vi "AutoBike FPGA (old).vi"() -> ()   [LabVIEW 2016]
doc: "The roboRIO FPGA Shipping Personality. This personality supports:\n- 8 Analog Input channels with 1 sample\n- 2 Analog Output channels with 1 sample\n- 30 Digital I/O channels with 1 sample\n- 1 RSL channel\n- 4 Relay channels\n- 1 Button\n- 3 LEDs\n- 1 Accelerometer\n- 13 PWM channels\n- 6 Encoder channels\n- 2 SPI channels\n- 2 I2C channels\n- 2 UART channels\n- 1 CAN channel\n- 2 Analog Input Interrupt\n- 5 Digital Input Interrupt\n- 1 Timer Interrupt"
uses:
  Sub VIs for FPGA/SubVIs needed for the customize FPGA VI/Utilities/Start Boolean.ctl
  <vilib>/rvi/Analysis/control/PID/Typedef/niFpgaPID_OutputRange.ctl
  <vilib>/rvi/Analysis/control/PID/Typedef/niFpgaPID_PIDGains.ctl
  <vilib>/rvi/Analysis/control/PID/Typedef/niFpgaPID_PIGains.ctl
  <vilib>/Platform/TimedLoop/XDataNode/timing_clust.ctl
  <vilib>/Platform/TimedLoop/XDataNode/nitl_modes.ctl
  <vilib>/Platform/TimedLoop/XDataNode/wakeup.ctl
  <vilib>/rvi/Analysis/control/PID/Typedef/niFpgaPID_SetpointWeightings.ctl
  <vilib>/rvi/Emulation/niFpgaGetClockAttributes.vi
  <vilib>/rvi/Emulation/niFpgaSctlEmulationGetInTimedLoop.vi
  <vilib>/rvi/Emulation/niFpgaEmulationReportErrorSimple.vi
  <vilib>/rvi/eio/common/nirviEmuTemplateMethod_errors.vi
  <vilib>/rvi/Emulation/niFpgaCriticalErrorInLSC.vi
  <vilib>/rvi/Emulation/niFpgaProcessEmulError.vi
  <vilib>/rvi/Emulation/niFpgaEmulationIsFPGAContextNoSignature.vi
  <vilib>/rvi/errors/niFpgaSetErrorForExecOnDevCompSimple.vi
  <vilib>/rvi/eio/common/nirviEmuReportErrorAndStop.vi
  <vilib>/rvi/DataTransferAndStorage/Container/Common/niFpgaContainerGetUniqueNameForEmu.vi
  <vilib>/rvi/FIFO/Fifo_Resource/nirvififoEmulationSetSize.vi
  <vilib>/rvi/FIFO/Fifo_Resource/nirviFifoEmulationQueueMgr.vi
  <instcachedir>/0/nirviFifoEmulationQueueMgr_E5CAEC123FF24DC58D834DCA3CDAA9B5.lvgen/nirviFifoEmulationQueueMgr_E5CAEC123FF24DC58D834DCA3CDAA9B5_002.vi
  <vilib>/Utility/error.llb/Clear Errors.vi
  <vilib>/rvi/FIFO/Fifo_Resource/nirvififoEmulationCreateLock.vi
  <vilib>/rvi/FIFO/Fifo_Resource/nirvififoEmulationObtainLock.vi
  <vilib>/rvi/FIFO/Fifo_Resource/nirvififoEmulationReleaseLock.vi
  <vilib>/rvi/occurrence/nirviWaitOnOccurrenceBase.vi
  <vilib>/rvi/errors/nirviReportUnexpectedCaseInternalError.vi
  <vilib>/rvi/errors/nirviReportUnexpectedCaseInternalError (U32).vi
  <vilib>/rvi/FIFO/Fifo_Resource/nirvififoEmulationDetermineInputValidOut.vi
  <vilib>/rvi/Analysis/control/PID/SubVIs/niFpgaPID_PIWrapper.vi
  <vilib>/rvi/Analysis/control/PID/SubVIs/niFpgaPID_PIDWrapper.vi
  <vilib>/rvi/DataTransferAndStorage/Container/Common/niFpgaContainerSetEmuInfo.vi
  <vilib>/eio/EIONode/EIONode.xnode
  <vilib>/rvi/DataTransferAndStorage/Container/XNode/niFpgaContainer.xnode
  <vilib>/rvi/FIFO/Fifo_Resource/nirvififoEmulationRead.vi
  <vilib>/rvi/FIFO/Fifo_Resource/nirvififoEmulationWrite.vi
  <vilib>/Platform/TimedLoop/XDataNode/XDataNode.xnode
  <vilib>/rvi/LocalResourceManager/LocalResourceManager.xnode
  <vilib>/Platform/TimedLoop/XDataNode/XDNodeRunTimeDep.lvlib
panel:
  out "Value Channel 3":i32
  out "Value Channel 2":i32
  in  "Speed output range":T1={"output high (Inf)"=0.0001, "output low (-Inf)"=-0.0001}
  in  "PI gains":T2={"proportional gain"=40.0, "integral gain"=15.0} {"proportional gain" step=0.125}
  out "Steering loop time":u32
  in  "Steering motor on?":bool
  in  "Gain Sch, on?":bool
  in  "Gain Sch.":T3[](array[typedef])=[{"proportional gain"=0.0, "integral gain"=0.0, "derivative gain"=0.0, "filter coefficient"=0.0}, {"proportional gain"=0.0, "integral gain"=0.0, "derivative gain"=0.0, "filter coefficient"=0.0}, {"proportional gain"=0.0, "integral gain"=0.0, "derivative gain"=0.0, "filter coefficient"=0.0}, {"proportional gain"=0.0, "integral gain"=0.0, "derivative gain"=0.0, "filter coefficient"=0.0}] {"filter coefficient" min=0 max=1; "proportional gain" step=0.125}
  in  "output range Sch.":T1[](array[typedef])=[{"output high (Inf)"=0.0, "output low (-Inf)"=0.0}, {"output high (Inf)"=0.0, "output low (-Inf)"=0.0}, {"output high (Inf)"=0.0, "output low (-Inf)"=0.0}, {"output high (Inf)"=0.0, "output low (-Inf)"=0.0}]
  in  "Desired steering angle":sgl format="%#_13g"
  in  "Stop PID controller":bool
  in  "Pid reset (F)":bool
  out "Current steering angle":sgl
  out "Duty cycle (steering)":sgl
  out "Position 2":i64
  in  "LQR Duty Cycle":sgl
  in  "LQR Direction":bool
  in  "Shut Down BW":bool
  out "Current speed":sgl
  out "Duty cycle (BW)":sgl
  in  "Reference speed in km/h":sgl=15.0
  out "Filtered data":i32
  out "Value Channel 0":i32
  out "Channel 4 position":u8
  out "Channel 5 position":u8
  out "Channel 6 position":u8
  out "Channel 7 position":u8
  out "Position":i32
  in  "Stop encoder":bool
  in  "Reset counter":bool
  in  "Stop direction switch":bool
  in  "Direction":bool
  out "HallSensorValue":u8
  out "dt":u32
  out "DIO.SPI_CS3:0.IN":u8 format="%08b"
  in  "DIO.SPI_CS3:0.DIR":u8 format="%08b"
  in  "DIO.SPI_CS3:0.OUT":u8 format="%08b"
  in  "IRQ.TIMER.SETTIME":T4
  in  "IRQ.TIMER.WRITE":u32
  out "IRQ.TIMER.READ":u32
  in  "IRQ.DI_BTN.NO":u8
  in  "IRQ.DI_BTN.CNT":u32
  in  "IRQ.DI_BTN.FALL":bool
  in  "IRQ.DI_BTN.RISE":bool
  in  "IRQ.DI_BTN.ENA":bool
  in  "IRQ.AI_B_0.HYSTERESIS":u16=17
  in  "IRQ.AI_B_1.HYSTERESIS":u16=17
  in  "IRQ.AI_B_1.NO":u8
  in  "IRQ.AI_B_0.NO":u8
  in  "IRQ.AI_B_1.THRESHOLD":u16
  in  "IRQ.AI_B_0.THRESHOLD":u16
  in  "IRQ.AI_B_3:0.CNFG":u8 format="%.0b"
  in  "IRQ.DIO_B_0.NO":u8
  in  "IRQ.DIO_B_1.NO":u8
  in  "IRQ.DIO_B_2.NO":u8
  in  "IRQ.DIO_B_3.NO":u8
  in  "IRQ.DIO_B_3.CNT":u32
  in  "IRQ.DIO_B_2.CNT":u32
  in  "IRQ.DIO_B_1.CNT":u32
  in  "IRQ.DIO_B_0.CNT":u32
  in  "IRQ.DIO_B_7:0.FALL":u8 format="%08b"
  in  "IRQ.DIO_B_7:0.RISE":u8 format="%08b"
  in  "IRQ.DIO_B_7:0.ENA":u8 format="%08b"
  in  "SPI.SPI.IRQ.NO":u8=15
  in  "SPI.B.IRQ.NO":u8=15
  out "DIO.DIO_9:8.IN":u8 format="%08b"
  in  "ENC.DIO_3.CNFG":u8 format="%08b"
  out "ENC.DIO_3.CNTR":u32
  out "ENC.DIO_3.STAT":u8 format="%08b"
  in  "ENC.DIO_4.CNFG":u8 format="%08b"
  out "ENC.DIO_4.CNTR":u32
  out "ENC.DIO_4.STAT":u8 format="%08b"
  in  "DIO.DIO_9:8.OUT":u8 format="%08b"
  in  "DIO.DIO_9:8.DIR":u8 format="%08b"
  in  "ENC.DIO_2.CNFG":u8 format="%08b"
  out "ENC.DIO_2.CNTR":u32
  out "ENC.DIO_2.STAT":u8 format="%08b"
  out "ENC.DIO_1.STAT":u8 format="%08b"
  out "ENC.DIO_1.CNTR":u32
  in  "ENC.DIO_1.CNFG":u8 format="%08b"
  out "DIO.DIO_7:0.IN":u8 format="%08b"
  in  "SYS.SELECTDIO":u8 format="%08b"
  in  "DIO.DIO_7:0.DIR":u8 format="%08b"
  in  "DIO.DIO_7:0.OUT":u8 format="%08b"
  out "ENC.DIO_0.STAT":u8 format="%08b"
  out "ENC.DIO_0.CNTR":u32
  in  "ENC.DIO_0.CNFG":u8 format="%08b"
  out "DI.BTN":u8 format="%08b"
  in  "DO.LED 5:0":u8 format="%06b"
  in  "DO.RSL.OUT":bool
  out "SPI.SPI.STAT":u8 format="%08b"
  in  "SPI.SPI.GO":T4
  in  "SPI.SPI.CNT":u16
  in  "SPI.SPI.CNFG":u16 format="%016b"
  out "SPI.SPI.DATI":u16
  in  "SPI.SPI.DATO":u16
  out "I2C.I2C.DATI":u8
  out "I2C.I2C.STAT":u8 format="%08b"
  in  "I2C.I2C.DATO":u8
  in  "I2C.I2CADDR":u8 format="%08b"
  in  "I2C.I2C.CNTR":u8
  in  "I2C.I2C.CNTL":u8 format="%08b"
  in  "I2C.I2C.CNFG":u8 format="%08b"
  in  "I2C.I2C.GO":T4
  out "ACC.Z.VAL":u16
  out "ACC.Y.VAL":u16
  out "ACC.X.VAL":u16
  in  "DO.RELAY.OUT":u8 format="%08b"
  out "SYS.ACC.RDY":bool
  out "SYS.RDY":bool
  in  "PWM.PWM_5.MAX":u16
  in  "PWM.PWM_5.CMP":u16
  in  "PWM.PWM_5.CNFG":u8 format="%08b"
  in  "PWM.PWM_5.CS":u8
  out "PWM.PWM_5.CNTR":u16
  in  "PWM.PWM_6.MAX":u16
  in  "PWM.PWM_6.CMP":u16
  in  "PWM.PWM_6.CNFG":u8 format="%08b"
  in  "PWM.PWM_6.CS":u8
  out "PWM.PWM_6.CNTR":u16
  in  "PWM.PWM_7.MAX":u16
  in  "PWM.PWM_7.CMP":u16
  in  "PWM.PWM_7.CNFG":u8 format="%08b"
  in  "PWM.PWM_7.CS":u8
  out "PWM.PWM_7.CNTR":u16
  in  "PWM.PWM_8.MAX":u16
  in  "PWM.PWM_8.CMP":u16
  in  "PWM.PWM_8.CNFG":u8 format="%08b"
  in  "PWM.PWM_8.CS":u8
  out "PWM.PWM_8.CNTR":u16
  in  "PWM.PWM_9.MAX":u16
  in  "PWM.PWM_9.CMP":u16
  in  "PWM.PWM_9.CNFG":u8 format="%08b"
  in  "PWM.PWM_9.CS":u8
  out "PWM.PWM_9.CNTR":u16
  in  "PWM.PWM_4.MAX":u16
  in  "PWM.PWM_4.CMP":u16
  in  "PWM.PWM_4.CNFG":u8 format="%08b"
  in  "PWM.PWM_4.CS":u8
  out "PWM.PWM_4.CNTR":u16
  in  "PWM.PWM_3.MAX":u16
  in  "PWM.PWM_3.CMP":u16
  in  "PWM.PWM_3.CNFG":u8 format="%08b"
  in  "PWM.PWM_3.CS":u8
  out "PWM.PWM_3.CNTR":u16
  in  "PWM.PWM_2.MAX":u16
  in  "PWM.PWM_2.CMP":u16
  in  "PWM.PWM_2.CNFG":u8 format="%08b"
  in  "PWM.PWM_2.CS":u8
  out "PWM.PWM_2.CNTR":u16
  in  "PWM.PWM_1.MAX":u16
  in  "PWM.PWM_1.CMP":u16
  in  "PWM.PWM_1.CNFG":u8 format="%08b"
  in  "PWM.PWM_1.CS":u8
  out "PWM.PWM_1.CNTR":u16
  out "PWM.PWM_0.CNTR":u16
  in  "PWM.PWM_0.CS":u8
  in  "PWM.PWM_0.CNFG":u8 format="%08b"
  in  "PWM.PWM_0.CMP":u16
  in  "PWM.PWM_0.MAX":u16
  in  "AO.B_0.VAL":u16
  in  "AO.B_1.VAL":u16
  in  "AO.SYS.GO":T4
  out "AO.SYS.STAT":bool
  out "AI.B_0.VAL":u16
  out "AI.B_1.VAL":u16
  out "AI.B_2.VAL":u16
  out "AI.B_3.VAL":u16
  out "AI.AI_0.VAL":u16
  out "AI.AI_1.VAL":u16
  out "AI.AI_2.VAL":u16
  out "AI.AI_3.VAL":u16
  out "SYS.AI.RDY":bool
  in  "SYS.SELECTB":u8 format="%08b"
  in  "DIO.B_7:0.OUT":u8 format="%08b"
  in  "DIO.B_7:0.DIR":u8 format="%08b"
  out "DIO.B_7:0.IN":u8 format="%08b"
  in  "DIO.B_15:8.OUT":u8 format="%08b"
  in  "DIO.B_15:8.DIR":u8 format="%08b"
  out "DIO.B_15:8.IN":u8 format="%08b"
  in  "SPI.B.DATO":u16
  out "SPI.B.DATI":u16
  in  "SPI.B.CNFG":u16 format="%016b"
  in  "SPI.B.CNT":u16
  in  "SPI.B.GO":T4
  out "SPI.B.STAT":u8 format="%08b"
  in  "PWM.B_0.MAX":u16
  in  "PWM.B_0.CMP":u16
  in  "PWM.B_0.CNFG":u8 format="%08b"
  in  "PWM.B_0.CS":u8
  out "PWM.B_0.CNTR":u16
  in  "PWM.B_1.CMP":u16
  in  "PWM.B_1.MAX":u16
  out "PWM.B_1.CNTR":u16
  in  "PWM.B_1.CNFG":u8 format="%08b"
  in  "PWM.B_1.CS":u8
  in  "PWM.B_2.CMP":u16
  in  "PWM.B_2.MAX":u16
  out "PWM.B_2.CNTR":u16
  in  "PWM.B_2.CNFG":u8 format="%08b"
  in  "PWM.B_2.CS":u8
  in  "I2C.B.DATO":u8
  out "I2C.B.DATI":u8
  in  "I2C.B.ADDR":u8 format="%08b"
  in  "I2C.B.CNTR":u8
  in  "I2C.B.CNTL":u8 format="%08b"
  out "I2C.B.STAT":u8 format="%08b"
  in  "I2C.B.CNFG":u8 format="%08b"
  in  "I2C.B.GO":T4
  in  "ENC.B.CNFG":u8 format="%08b"
  out "ENC.B.CNTR":u32
  out "ENC.B.STAT":u8 format="%08b"
  # "System"
  # "Onboard Devices"
  # "Connector B"
  # "DIO"
  # "SPI"
  # "PWM"
  # "I2C"
  # "AI"
  # "RELAY"
  # "RSL"
  # "Accelerometer"
  # "SPI Master"
  # "Analog Input"
  # "Analog Output"
  # "Digital I/O"
  # "Counters / PWM"
  # "Digital I/O"
  # "Encoders"
  # "IO Configuration"
  # "Buttons & LEDs"
  # "SPI CS DIO"
  # "Analog Interrupt"
  # "Digital Interrupt"
  # "Encoders"
  # "IO Configuration"
  # "Button Interrupt"
  # "I2C Master"
  # "FPGA Timer"
types:
  T1 = typedef "niFpgaPID_OutputRange.ctl" = cluster{"output high (Inf)":sgl, "output low (-Inf)":sgl}
  T2 = typedef "niFpgaPID_PIGains.ctl" = cluster{"proportional gain":sgl, "integral gain":sgl}
  T3 = typedef "niFpgaPID_PIDGains.ctl" = cluster{"proportional gain":sgl, "integral gain":sgl, "derivative gain":sgl, "filter coefficient":sgl}
  T4 = typedef "Start Boolean.ctl" = bool
  T5 = typedef "XDNodeRunTimeDep.lvlib/timing_clust.ctl" = cluster{"Expected End [f-1]":u64, "Actual End [f-1]":u64, "Finished Late? [f-1]":bool, "Expected End [i-1]":u64, "Actual End [i-1]":u64, "Finished Late? [i-1]":bool, "Expected Start [i]":u64, "Actual Start [i]":u64, "Expected Start [f]":u64, "Actual Start [f]":u64, "Source Name":string, "Structure Name":string, "Period":i64, "Deadline":i64, "Offset":i64, "Start":i64, "Priority":i32, "Timeout":i32, "Mode":T6, "Wakeup Reason":T7, "Error":errorcluster, "Source Type":string, "Secondary Source Type":string, "Global End Time":u64, "Global Start Time":u64, "Frame Duration":u64, "Iteration Duration":u64, "Assigned CPU":i32, "I/O Scan Engine Mode":u32}
  T6 = typedef "XDNodeRunTimeDep.lvlib/nitl_modes.ctl" = enum32{"No Change", "Process missed periods, maintain original phase", "Discard missed periods, maintain original phase", "Process missed periods, ignore original phase", "Discard missed periods, ignore original phase"}
  T7 = typedef "XDNodeRunTimeDep.lvlib/wakeup.ctl" = enum32{"Normal", "Aborted", "Asynchronous wakeup", "Timing source error", "Timed loop error", "Timeout"}
  T8 = typedef "niFpgaPID_SetpointWeightings.ctl" = cluster{"proportional weighting (1)":sgl, "derivative weighting (0)":sgl}
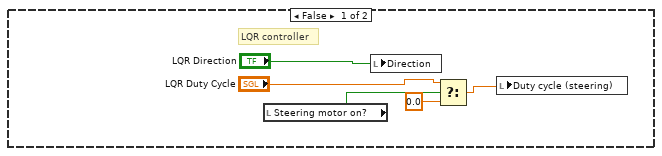
[diagram p8: hidden frame]
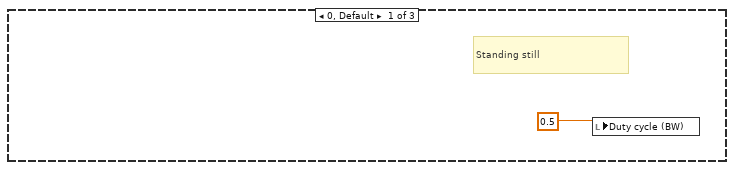
[diagram p9: hidden frame]
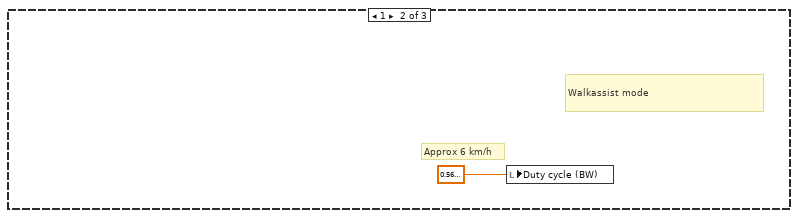
[diagram p10: hidden frame]
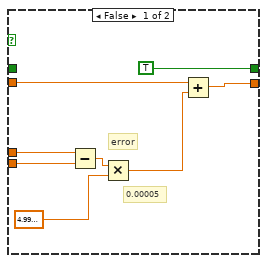
[diagram p11: hidden frame]
diagram:
  # "Runs at 40 MHz"
  # "The accelerometer nodes take some time before the FPGA can first read the values. This is because it takes time to read from the accelerometer. An iteration of the While Loop will not complete until the accelerometer values have been read.\n\nAfter the completion of the first iteration of the While Loop, all indicators have valid values."
  # "The analog output nodes take some time before the FPGA write the values to the pins. The GO and STAT registers are used to handshake between the FPGA and host. When the host wants the values to be written, the host sets the GO register to TRUE. If the host reads the STAT register before setting the value of the GO register, it can wait for the value of the STAT register to invert. The value inversion tells the host that the output values have been written."
  # "The FPGA timer fires the interrupt request (IRQ) when TIMER.Read counts down to zero. If TIMER.Read is not zero, it counts down to one per microsecond."
  # "The analog input nodes take some time before the FPGA can first read the values. This is because it takes time to set up the Analog-to-Digital converter (ADC) and convert the first reading. An iteration of the While Loop will not complete until all the analog input channels have been sampled.\n\nAfter the completion of the first iteration of the While Loop, all indicators have valid values."
  # "Note: On some hardware a \"ghosting effect\" may occur on any unconnected AI channels. For example, if channel AI0 is connected and channels AI1~AI7 are not connected the the value read at AI0 may be seen on indicators AI1~AI7. This is common for hardware that use a multiplexed (MUXed) Analog-to-Digital converter (ADC), because the input analog signal is used to charge a capacitor which does not discharge before the unconnected channel is read.\n\nYou can hide the \"ghosting effect\" by using an mask register. This register is used to decide when the indicator should be updated."
  # "The only interface that sends interrupts to the RT side. Timer interrupts, analog input interrupts, digital input interrupts, and SPI interrupt share this interface.\n\nAll interrupts work in sequence. One interrupt waits until the previous interrupt request (IRQ) gets acknowledged on the RT side."
  # "NOTE: The SYS.RDY boolean MUST exist and must become TRUE at some point otherwise the myRIO API will not function correctly."
  # "There is some delay between when the FPGA code starts and the analog inputs, accelerometer, and scaling values outputs are valid. If the host wants to ensure that there are valid values in theses registers it should wait for each subsystem to finish its initialization process. \n\nWhen all subsystems have finished initializinig, the SYS.RDY indicator will be true, which can be polled by the host to determine the status of the FPGA. Alternatively, the host can poll the individual SYS.xx.RDY indicators to determine the status of the individual subsystems.\n\nThis loop continues indefinitely, essentially making SYS.RDY a read-only register."
  n1 = while {
    shift-right: [w32] -> _
    shift-left: TRUE ("DIO/DIO3") -> [w33]
    stop <- FALSE stop-if-true
    n2 = flat-sequence {
      tunnel: w33 -> [w36]
      tunnel: [w36] -> w31
      tunnel: [u8 0] -> w30
      tunnel: [w34] -> w29
      tunnel: w31 -> [w41]
      tunnel: w30 -> [w39]
      tunnel: w29 -> [w38]
      tunnel: [w40] -> w28
      tunnel: [w37] -> w27
      tunnel: [w63] -> w32
      tunnel: w28 -> [w63]
      tunnel: [w62] -> w26
      tunnel: w27 -> [w60]
      frame #0 {
        n3 = call "Tick Count4"() -> ("Tick Count(uSec)"=w34:u32)
      }
      frame #1 {
        n4 = node-c288() -> (w43:T5)  [unwired: 1 in]
        n5 = timed-loop {
          shift-right: [w44] -> _
          shift-left: w39 -> [w45]
          shift-right: [w52] -> w40
          shift-left: w41 -> [w55]
          timing: w43 -> [_]
          timing-out: [_] -> w42
          tunnel: w38 -> [w54]
          tunnel: [w54] -> w37
          stop <- w47 stop-if-true
          # "Calculates the time it takes to collect 2 rises, i.e one magnet"
          # "Reads the output from the hallsensor and outputs the number of change in rises"
          # "Hallsensor counter"
          n6 = xnode "FPGA I/O Node"() -> ("DIO/DIO8"=w52:bool)  [unwired: 1 in, 1 out]
          n7 = Exclusive Or(1:w55, 2:w52) -> (0:w50:bool)
          n8 = Not And(1:TRUE ("y"), 2:w52) -> (0:w51:bool)
          n9 = And(x=w51, y=w50) -> (x .and. y?=w49:bool)
          n10 = Increment(x=w45) -> (x+1=w48:u8)
          n11 = Select(t=w48, s=w49, f=w45) -> (s? t:f=w44:u8)
          "HallSensorValue" <- w44
          n12 = Equal?(x=u8 2, y=w44) -> (x = y?=w47:bool)
        }
        n13 = node-c288(w42) -> ()
      }
      frame #2 {
        n14 = call "Tick Count"() -> ("Tick Count(uSec)"=w61:u32)
        n15 = Subtract(x=w61, y=w60) -> (x-y=w62:u32)
      }
    }
    n16 = To Long Integer(number=w26) -> (32bit integer=w25:i32)
    n17 = call "Median filter.vi"("Rawdata"=w25) -> ("Filtered element"=w22:i32)  [unwired: 10 in]
    n18 = Equal To 0?(x=w22) -> (x = 0?=w24:bool)
    n19 = Select(t=1, s=w24, f=w22) -> (s? t:f=→"Filtered data":i32)
  }
  n20 = node-c288() -> (w8:T5)  [unwired: 1 in]
  n21 = while {
    stop <- FALSE stop-if-true
    # "PWM signal to backwheel motor"
    n22 = flat-sequence {
      tunnel: [w69] -> w65
      tunnel: w65 -> [w72]
      frame #0 {
        # "80 000ticks=500Hz"
        n23 = call "Loop Timer2"("Count(Ticks)"=u32 80000) -> ()  [unwired: 1 out]
      }
      frame #1 {
        n24 = local read "Duty cycle (BW)"() -> (w67:sgl)
        n25 = xnode "FPGA I/O Node"("PWM/PWM8"=TRUE) -> ()  [unwired: 1 in, 1 out]
        n26 = Multiply(x=w67, y=sgl 80000.0) -> (x*y=w70:sgl)
        n27 = To Unsigned Long Integer(number=w70) -> (unsigned 32bit integer=w69:u32)
      }
      frame #2 {
        n28 = call "Wait2"("Count(Ticks)"=w72) -> ()  [unwired: 1 out]
      }
      frame #3 {
        n29 = xnode "FPGA I/O Node"("PWM/PWM8"=FALSE) -> ()  [unwired: 1 in, 1 out]
      }
    }
  }
  n30 = node-c288() -> (w6:T5)  [unwired: 1 in]
  n31 = while {
    stop <- FALSE stop-if-true
    # "Host Synchronization"
    n32 = local read "SYS.ACC.RDY"() -> (w75:bool)
    n33 = local read "SYS.AI.RDY"() -> (w77:bool)
    n34 = Compound Arithmetic op=AND(w77, w75) -> (→"SYS.RDY":bool)
  }
  n35 = timed-loop {
    shift-right: [w88] -> _
    shift-left: 0 -> [w79]
    shift-right: [w85] -> _
    shift-left: _ -> [w83]
    shift-right: [w84] -> _
    shift-left: _ -> [w82]
    timing: w8 -> [_]
    timing-out: [_] -> w7
    stop <- "Stop encoder" stop-if-true
    # "Decoder, reads both signals and check if there is any change to any of the channels, if there is a change current A channel\nis compared to previous B channel to determine which direction the motor is going and updates the position counter\naccordingly. The counter is resetted each time the Main VI is deployed."
    # "Steering motor decoder"
    n36 = xnode "FPGA I/O Node"() -> ("DIO/DIO0"=w85:bool, "DIO/DIO1"=w84:bool)  [unwired: 2 in, 2 out]
    n37 = Exclusive Or(1:w82, 2:w85) -> (0:w81:bool)
    n38 = Select(t=0, s="Reset counter", f=w79) -> (s? t:f=w87:i32)
    n39 = Exclusive Or(1:w83, 2:w85) -> (0:w95:bool)
    n40 = Exclusive Or(1:w82, 2:w84) -> (0:w94:bool)
    n41 = Or(x=w95, y=w94) -> (x .or. y?=w80:bool)
    n42 = Select(t=1, s=w81, f=-1) -> (s? t:f=w90:i32)
    n43 = Add(x=w90, y=w87) -> (x+y=w89:i32)
    n44 = Select(t=w89, s=w80, f=w87) -> (s? t:f=w88:i32)
    "Position" <- w88
  }
  n45 = timed-loop {
    timing: w6 -> [_]
    timing-out: [_] -> w5
    stop <- "Stop direction switch" stop-if-true
    # "Switch the direction of the steering\nmotor."
    # "Switch direction"
    n46 = xnode "FPGA I/O Node"("DIO/DIO2"="Direction") -> ()  [unwired: 1 in, 1 out]
  }
  n47 = while {
    stop <- FALSE stop-if-true
    # "PWM signal to steering motor"
    n48 = flat-sequence {
      tunnel: [w105] -> w102
      tunnel: [w110] -> w104
      tunnel: w102 -> [w107]
      tunnel: w104 -> [w112]
      frame #0 {
        w105 = u32 40000 ("Freq")
        # "40000 ticks=1kHz"
        n49 = call "Loop Timer3"("Count(Ticks)"=w105) -> ()  [unwired: 1 out]
      }
      frame #1 {
        # "Too make sure 0 duty \ncycle is generated"
        n50 = local read "Duty cycle (steering)"() -> (w108:sgl)
        n51 = To Single Precision Float(number=w107) -> (single precision float=w106:sgl)
        n52 = Not Equal To 0?(x=w108) -> (x != 0?=w109:bool)
        n53 = Multiply(x=w108, y=w106) -> (x*y=w111:sgl)
        n54 = xnode "FPGA I/O Node"("PWM/PWM0"=w109) -> ()  [unwired: 1 in, 1 out]
        n55 = To Unsigned Long Integer(number=w111) -> (unsigned 32bit integer=w110:u32)
      }
      frame #2 {
        n56 = call "Wait3"("Count(Ticks)"=w112) -> ()  [unwired: 1 out]
      }
      frame #3 {
        n57 = xnode "FPGA I/O Node"("PWM/PWM0"=FALSE ("PWM/PWM8")) -> ()  [unwired: 1 in, 1 out]
      }
    }
  }
  n58 = while {
    stop <- FALSE stop-if-true
    # "Convert Hall sensor pulses to current speed"
    n59 = local read "Filtered data"() -> (w115:i32)
    n60 = call "Speed conversion.vi"("Filtered data"=w115) -> ("Numeric"=→"Current speed":sgl)  [unwired: 10 in]
  }
  n61 = node-c288(w5) -> ()
  n62 = while {
    stop <- FALSE stop-if-true
    # "Backwheel motor control"
    n63 = local read "Channel 5 position"() -> (w117:u8)
    n64 = case shown="2" w117 {
      frame 0, Default {
        # "Standing still"
        n65 = local write "Duty cycle (BW)"(sgl 0.5 ("Duty cycle out 2")) -> ()
      }
      frame 1 {
        # "Walkassist mode"
        # "Approx 6 km/h"
        n66 = local write "Duty cycle (BW)"(sgl 0.56 ("Duty cycle out")) -> ()
      }
      frame 2 {
        n67 = while {
          shift-right: [w125] -> _
          shift-left: sgl 0.56 -> [w135]
          shift-right: [w134] -> _
          shift-left: _ -> [w133]
          stop <- w136 stop-if-true
          w124 = sgl 3.0 ("upper limit")
          # "P or PI controller"
          # "Cruise control"
          n68 = local read "Current speed"() -> (w123:sgl)
          n69 = Subtract(x="Reference speed in km/h", y=w123) -> (x-y=w131:sgl)
          n70 = Negate(x=w124) -> (-x=w129:sgl)
          n71 = In Range and Coerce(upper limit=w124, x=w131, lower limit=w129) -> (In Range?=w130:bool)  [unwired: 1 out]
          n72 = case shown="True" w130 {
            tunnel: [w146 w155] -> w128
            tunnel: "Reference speed in km/h" -> [w142 w153]
            tunnel: w135 -> [w144 w154]
            tunnel: w123 -> [w141 w152]
            tunnel: [TRUE FALSE] -> w134
            tunnel: w133 -> [_ w147]
            frame False {
              # "error"
              # "0.00005"
              n73 = Subtract(x=w142, y=w141) -> (x-y=w143:sgl)
              n74 = Multiply(x=w143, y=sgl 5e-05 ("P gain")) -> (x*y=w145:sgl)
              n75 = Add(x=w144, y=w145) -> (x+y=w146:sgl)
            }
            frame True {
              # "Gains"
              # "Output range"
              n76 = call-poly <vilib>:"niFpgaPID_Wrapper.vi"("setpoint"=w153, "reset? (F)"=w147, "process variable"=w152, "gains"="PI gains", "output range"="Speed output range") -> ("output"=w151:sgl)  [unwired: 8 in, 2 out]
              n77 = Add(x=w154, y=w151) -> (x+y=w155:sgl)
            }
          }
          n78 = local read "Channel 5 position"() -> (w138:u8)
          n79 = In Range and Coerce(upper limit=sgl 1.0, x=w128, lower limit=sgl 0.565) -> (coerced(x)=w125:sgl)  [unwired: 1 out]
          "Duty cycle (BW)" <- w125
          n80 = Not Equal?(x=w138, y=u8 2) -> (x != y?=w136:bool)
          n81 = call "Loop Timer5"("Count(Ticks)"=u32 400000 ("Speed loop time")) -> ()  [unwired: 1 out]
        }
      }
    }
  }
  n82 = while {
    stop <- FALSE stop-if-true
    # "Interrupt to RT"
    n83 = xnode ("FIFO Method Node")("Timeout"=-1) -> ("Element"=w158:u8)  [unwired: 1 in, 2 out]
    n84 = call <vilib>:"niFPGA Interrupt.vi"("Wait Until Cleared (F)"=TRUE, "IRQ Number (0)"=w158) -> ()  [unwired: 1 in]
  }
  n85 = while {
    stop <- FALSE stop-if-true
    # "RC steering motor switch"
    n86 = local read "Channel 6 position"() -> (w161:u8)
    n87 = Greater Than 0?(x=w161) -> (x > 0?=w160:bool)
    n88 = case shown="True" w160 {
      frame False {
        # "LQR controller"
        n89 = local read "Steering motor on?"() -> (w164:bool)
        n90 = local write "Direction"("LQR Direction") -> ()
        n91 = Select(t="LQR Duty Cycle", s=w164, f=sgl 0.0) -> (s? t:f=w165:sgl)
        n92 = local write "Duty cycle (steering)"(w165) -> ()
      }
      frame True {
        # "Control loop"
        n93 = while {
          shift-right: [w172] -> _
          shift-left: u32 0 ("Tick Count(Ticks)") -> [w173]
          stop <- w183 stop-if-true
          n94 = local read "Position"() -> (w186:i32)
          n95 = To Single Precision Float(number=w186) -> (single precision float=w185:sgl)
          n96 = call "Tick Count2"() -> ("Tick Count(Ticks)"=w172:u32)
          n97 = call "Loop Timer4"("Count(Ticks)"=u32 66666 ("loop wait time (ticks)")) -> ()  [unwired: 1 out]
          n98 = Divide(x=w185, y=sgl 616.667) -> (x/y=w170:sgl)
          "Current steering angle" <- w170
          n99 = Subtract(x=w172, y=w173) -> (x-y=→"Steering loop time":u32)
          n100 = local read "Channel 6 position"() -> (w181:u8)
          n101 = call-poly <vilib>:"niFpgaPID_Wrapper.vi"("setpoint"="Desired steering angle", "reset? (F)"="Pid reset (F)", "process variable"=w170, "gains"=T3 {"proportional gain"=0.1, "integral gain"=0.0, "derivative gain"=0.04, "filter coefficient"=0.8}, "output range"=T1 {"output high (Inf)"=0.5, "output low (-Inf)"=-0.5}, "setpoint weighting"=T8 {"proportional weighting (1)"=1.0, "derivative weighting (0)"=0.0}) -> ("output"=w188:sgl)  [unwired: 7 in, 2 out]
          n102 = Absolute Value(x=w188) -> (abs(x)=w177:sgl)
          n103 = Greater Than 0?(x=w188) -> (x > 0?=w178:bool)
          n104 = Select(t=w177, s="Steering motor on?", f=sgl 0.0) -> (s? t:f=→"Duty cycle (steering)":sgl)
          n105 = Not Equal?(x=w181, y=u8 1) -> (x != y?=w179:bool)
          n106 = local write "Direction"(w178) -> ()
          n107 = Or(x=w179, y="Stop PID controller") -> (x .or. y?=w183:bool)
        }
      }
    }
  }
  n108 = node-c288(w7) -> ()
  n109 = while {
    stop <- FALSE stop-if-true
    # "Receiver"
    n110 = call "Receiver.vi"() -> ("Channel 7 position"=→"Channel 7 position":u8, "Channel 6 position"=→"Channel 6 position":u8, "Channel 5 position"=w198:u8, "Channel 4 position"=→"Channel 4 position":u8, "Value Channel 0"=→"Value Channel 0":i32, "Value Channel 2"=→"Value Channel 2":i32, "Value Channel 3"=→"Value Channel 3":i32)  [unwired: 5 in]
    n111 = Select(t=u8 0, s="Shut Down BW", f=w198) -> (s? t:f=→"Channel 5 position":u8)
  }
  n112 = disable-structure shown="Disabled" {
    frame Disabled {
      n113 = while {
        stop <- FALSE stop-if-true
        # "Gain scheduler"
        n114 = case shown="True" "Gain Sch, on?" {
          tunnel: "Gain Sch." -> [_ w213]
          tunnel: "output range Sch." -> [_ w211]
          frame False {
          }
          frame True {
            w229 = sgl 20.0 ("upper limit")
            w230 = sgl 10.0 ("upper limit")
            w231 = sgl 3.0 ("upper limit")
            n115 = local read item#-1() -> (w234)
            n116 = Absolute Value(x=w234) -> (abs(x)=w233:dbl)
            n117 = In Range and Coerce(upper limit=w229, x=w233, lower limit=w230) -> (In Range?=w217:bool)  [unwired: 1 out]
            n118 = In Range and Coerce(upper limit=w230, x=w233, lower limit=w231) -> (In Range?=w218:bool)  [unwired: 1 out]
            n119 = In Range and Coerce(upper limit=w231, x=w233, lower limit=sgl 0.0) -> (In Range?=w219:bool)  [unwired: 1 out]
            n120 = In Range and Coerce(upper limit=sgl inf, x=w233, lower limit=w229) -> (In Range?=w216:bool)  [unwired: 1 out]
            n121 = Build Array(w217, w216) -> (w215:bool[])
            n122 = Or(x=w216, y=w217) -> (x .or. y?=w225:bool)
            n123 = Build Array(w219, w218) -> (w214:bool[])
            n124 = Boolean Array To Number(Boolean array=w215) -> (number=w224:u8)
            n125 = Boolean Array To Number(Boolean array=w214) -> (number=w226:u8)
            n126 = Add(x=u32 2, y=w224) -> (x+y=w222:u32)
            n127 = Select(t=w222, s=w225, f=u32 0) -> (s? t:f=w220:u32)
            n128 = Add(x=w220, y=w226) -> (x+y=w210:u32)
            n129 = Decrement(x=w210) -> (x-1=w227:u32)
            n130 = Decrement(x=w210) -> (x-1=w212:u32)
            n131 = Index Array(array=w213, index=w227) -> (element=w208:T3)
            n132 = Index Array(array=w211, index=w212) -> (element=w209:T1)
            n133 = local write item#-1(w209) -> ()
            n134 = local write item#-1(w208) -> ()
          }
        }
      }
    }
    frame Enabled {
    }
  }
  n135 = while {
    stop <- FALSE stop-if-true
    # "10Hz"
    # "Gaspedal"
    n136 = local read "Value Channel 2"() -> (w236:i32)
    n137 = local read "Channel 5 position"() -> (w237:u8)
    n138 = call "Loop Timer6"("Count(mSec)"=u16 100) -> ()  [unwired: 1 out]
    n139 = call "Throttle function FPGA.vi"("RC input"=w236, "Channel 5 position"=w237) -> ("Reference velocity"=w238:sgl)  [unwired: 9 in]
    n140 = local write "Reference speed in km/h"(w238) -> ()
  }
  n141 = while {
    stop <- FALSE stop-if-true
    # "Timer"
    n142 = local read "IRQ.TIMER.READ"() -> (w243:u32)
    n143 = Select(t="IRQ.TIMER.WRITE", s="IRQ.TIMER.SETTIME", f=w243) -> (s? t:f=w241:u32)
    n144 = case shown="Default" w241 {
      selector: w241 -> [w247 w250]
      tunnel: [w247 w248] -> w240
      frame 0 {
      }
      frame Default {
        n145 = Decrement(x=w250) -> (x-1=w249:u32)
        n146 = case shown="0" w249 {
          selector: w249 -> [w251 w254]
          tunnel: [w251 w254] -> w248
          frame Default {
          }
          frame 0 {
            w253 = u8 0  # Reserved for Timer IRQ
            n147 = xnode ("FIFO Method Node")("Element"=w253, "Timeout"=-1) -> ()  [unwired: 1 in, 2 out]
          }
        }
      }
    }
    "IRQ.TIMER.READ" <- w240
    n148 = call "Loop Timer"("Count(uSec)"=u8 1 ("Count(mSec)")) -> ()  [unwired: 1 out]
  }
  n149 = xnode "VI-Defined FIFO Configuration"() -> ("FIFO Out"=w1:refnum<k21>)
  n150 = while {
    tunnel: w1 -> [w263]
    i -> [w277]
    stop <- FALSE stop-if-true
    # "Analog Input"
    n151 = Greater Than 0?(x=w277) -> (x > 0?=→"SYS.AI.RDY":bool)
    n152 = xnode "FPGA I/O Node"() -> ("MXP/AI0"=w256:u16, "MXP/AI1"=w255:u16, "MXP/AI2"=→"AI.B_2.VAL":u16, "MXP/AI3"=→"AI.B_3.VAL":u16, "AnalogIn0"=→"AI.AI_0.VAL":u16, "AnalogIn1"=→"AI.AI_1.VAL":u16, "AnalogIn2"=→"AI.AI_2.VAL":u16, "AnalogIn3"=→"AI.AI_3.VAL":u16)  [unwired: 8 in, 8 out]
    "AI.B_0.VAL" <- w256
    "AI.B_1.VAL" <- w255
    n153 = Number To Boolean Array(number="IRQ.AI_B_3:0.CNFG") -> (Boolean array=w264:bool[])
    n154 = Index Array(array=w264) -> (element #1=w266:bool, element #2=w267:bool, element #3=w269:bool, element #4=w270:bool)  [unwired: 4 in]
    n155 = call "Check AI IRQ.vi"("Hysteresis"="IRQ.AI_B_1.HYSTERESIS", "FIFO In"=w263, "IRQ Number"="IRQ.AI_B_1.NO", "Threshold"="IRQ.AI_B_1.THRESHOLD", "Analog Value"=w255, "Rising Edge?"=w270, "Enable Interrupt?"=w269) -> ()  [unwired: 5 in]
    n156 = call "Check AI IRQ.vi"("Hysteresis"="IRQ.AI_B_0.HYSTERESIS", "FIFO In"=w263, "IRQ Number"="IRQ.AI_B_0.NO", "Threshold"="IRQ.AI_B_0.THRESHOLD", "Analog Value"=w256, "Rising Edge?"=w267, "Enable Interrupt?"=w266) -> ()  [unwired: 5 in]
  }
  n157 = while {
    stop <- FALSE stop-if-true
    # "Analog Output"
    n158 = feedback #1(FALSE) -> (w281:bool)
    n159 = case shown="True" "AO.SYS.GO" {
      tunnel: "AO.B_0.VAL" -> [_ w291]
      tunnel: "AO.B_1.VAL" -> [_ w290]
      tunnel: w281 -> [w286 w289]
      tunnel: [w286 w287] -> w279
      frame False {
      }
      frame True {
        n160 = flat-sequence {
          tunnel: w291 -> [w294]
          tunnel: w290 -> [w293]
          tunnel: w289 -> [w292]
          tunnel: [w292] -> w288
          tunnel: w288 -> [w296]
          tunnel: [w295] -> w287
          frame #0 {
            n161 = xnode "FPGA I/O Node"("MXP/AO0"=w294, "MXP/AO1"=w293) -> ()  [unwired: 2 in, 2 out]
          }
          frame #1 {
            n162 = Not(x=w296) -> (.not. x?=w295:bool)
          }
        }
      }
    }
    "AO.SYS.STAT" <- w279
    n163 = feedback-in #1(w279) -> ()
  }
  n164 = while {
    i -> [w304]
    stop <- FALSE stop-if-true
    # "Onboard Accelerometer"
    n165 = xnode "FPGA I/O Node"() -> ("AccelerationX"=w302:i16, "AccelerationY"=w301:i16, "AccelerationZ"=w300:i16)  [unwired: 3 in, 3 out]
    n166 = Greater Than 0?(x=w304) -> (x > 0?=→"SYS.ACC.RDY":bool)
    n167 = To Unsigned Word Integer(number=w302) -> (unsigned 16bit integer=→"ACC.X.VAL":u16)
    n168 = To Unsigned Word Integer(number=w301) -> (unsigned 16bit integer=→"ACC.Y.VAL":u16)
    n169 = To Unsigned Word Integer(number=w300) -> (unsigned 16bit integer=→"ACC.Z.VAL":u16)
  }
  n170 = xnode "VI-Defined FIFO Configuration"() -> ("FIFO Out"=w11:refnum<k21>)
  n171 = node-c288() -> (w15:T5)  [unwired: 1 in]
  n172 = timed-loop {
    timing: w15 -> [_]
    timing-out: [_] -> w14
    tunnel: w11 -> [w311]
    stop <- FALSE stop-if-true
    # "Button IRQ"
    # "Onboard DIO"
    n173 = xnode "FPGA I/O Node"() -> ("User Button"=w312:bool)  [unwired: 1 in, 1 out]
    n174 = Number To Boolean Array(number="DO.LED 5:0") -> (Boolean array=w322:bool[])
    n175 = Index Array(array=w322) -> (element #1=w320:bool, element #2=w319:bool, element #3=w318:bool, element #4=w317:bool, element #5=w316:bool, element #6=w315:bool)  [unwired: 6 in]
    n176 = Build Array(w312) -> (w314:bool[])
    n177 = call "DIO IRQ 1-bit.vi"("IRQ.NO"="IRQ.DI_BTN.NO", "IRQ.CNT"="IRQ.DI_BTN.CNT", "FIFO in"=w311, "IRQ.FALL"="IRQ.DI_BTN.FALL", "IRQ.RISE"="IRQ.DI_BTN.RISE", "IRQ.ENA"="IRQ.DI_BTN.ENA", "DIO"=w312) -> ()  [unwired: 5 in]
    n178 = Boolean Array To Number(Boolean array=w314) -> (number=→"DI.BTN":u8)
    n179 = xnode "FPGA I/O Node"("Radio LED Green"=w320, "Radio LED Red"=w319, "Comm LED Green"=w318, "Comm LED Red"=w317, "Mode LED Green"=w316, "Mode LED Red"=w315) -> ()  [unwired: 6 in, 6 out]
  }
  n180 = while {
    stop <- FALSE stop-if-true
    # "Button SCTL Interrupt Buffer"
    n181 = feedback #2(u8 0 ("Element")) -> (w328:u8)
    n182 = feedback #3(FALSE ("Timed Out?")) -> (w332:bool)
    n183 = case shown="False" w332 {
      tunnel: [w334 w336] -> w329
      tunnel: w328 -> [_ w336]
      frame False {
        n184 = xnode ("FIFO Read")("Timeout"=-1) -> ("Element"=w334:u8)  [unwired: 1 in, 2 out]
      }
      frame True {
      }
    }
    n185 = feedback-in #2(w329) -> ()
    n186 = xnode ("FIFO Method Node")("Element"=w329, "Timeout"=0) -> ("Timed Out?"=w330:bool)  [unwired: 1 in, 1 out]
    n187 = feedback-in #3(w330) -> ()
  }
  n188 = node-c288(w14) -> ()
  n189 = xnode "VI-Defined FIFO Configuration"() -> ("FIFO Out"=w13:refnum<k21>)
  n190 = xnode "VI-Defined FIFO Configuration"() -> ("FIFO Out"=w12:refnum<k21>)
  n191 = node-c288() -> (w19:T5)  [unwired: 1 in]
  n192 = timed-loop {
    timing: w19 -> [_]
    timing-out: [_] -> w18
    tunnel: w13 -> [w373]
    tunnel: w12 -> [w361]
    stop <- _ stop-if-true
    # "DIO/ IRQ"
    # "DIO / Encoder"
    # "DIO / I2C Master"
    # "DIO / PWM"
    # "DIO"
    # "DIO"
    # "DIO/ SPI Master"
    # "Connector MXP DIO"
    n193 = call "Split HDC Bank1 DIO.vi"("IN 7:0"="DIO.B_7:0.OUT") -> ("OUT 3:0"=w461:fxp<+,4,4>, "OUT 4"=w376:bool, "OUT 7:5"=w458:fxp<+,3,3>)
    n194 = call "Split HDC Bank1 DIO.vi"("IN 7:0"="DIO.B_7:0.DIR") -> ("OUT 3:0"=w460:fxp<+,4,4>, "OUT 4"=w459:bool, "OUT 7:5"=w457:fxp<+,3,3>)
    n195 = call "Split HDC Function Select.vi"("IN 7:0"="SYS.SELECTB") -> ("OUT 1:0"=w397:fxp<+,2,2>, "OUT 7"=w392:bool, "OUT 2"=w396:bool, "OUT 3"=w395:bool, "OUT 4"=w394:bool, "OUT 5"=w393:bool)
    n196 = call "DIO 4-bit.vi"("DIO0 Refnum"=refnum<k21> "MXP/DIO0", "DIO1 Refnum"=refnum<k21> "MXP/DIO1", "DIO2 Refnum"=refnum<k21> "MXP/DIO2", "DIR 3:0"=w460, "OUT 3:0"=w461, "DIO3 Refnum"=refnum<k21> "MXP/DIO3") -> ("IN 3:0"=w372:fxp<+,4,4>)  [unwired: 5 in]
    n197 = call "DIO 1-bit.vi"("DIR"=w459, "OUT"=w376, "DIO Refnum"=refnum<k21> "MXP/DIO4") -> ("IN"=w433:bool)  [unwired: 8 in]
    n198 = call "DIO_SPI.vi"("DIO.2:0.OUT"=w458, "DIO.2:0.DIR"=w457, "SPI.CNT"="SPI.B.CNT", "SPI.CNFG"="SPI.B.CNFG", "SPI.DATO"="SPI.B.DATO", "SPI.GO"="SPI.B.GO", "DIO.2/SPI.MOSI Refnum"=refnum<k21> "MXP/DIO7" ("DIO.2/SPI.SCLK"), "SELECT.1:0"=w397, "DIO.1/SPI.MISO Refnum"=refnum<k21> "MXP/DIO6" ("DIO.1/SPI.MOSI"), "DIO.0/SPI.SCLK Refnum"=refnum<k21> "MXP/DIO5" ("DIO.0/SPI.MISO")) -> ("DIO.2:0.IN"=w432:fxp<+,3,3>, "SPI.DATI"=→"SPI.B.DATI":u16, "SPI.STAT"=w375:u8)  [unwired: 7 in]
    "SPI.B.STAT" <- w375
    n199 = call "SPI IRQ.vi"("SPI.A.IRQ.NO"="SPI.B.IRQ.NO", "SPI.STAT"=w375, "FIFO In"=w373) -> ()  [unwired: 9 in]
    n200 = call "Join HDC Bank1 DIO.vi"("IN 7:5"=w432, "IN 4"=w433, "IN 3:0"=w372) -> ("OUT 7:0"=→"DIO.B_7:0.IN":u8)
    n201 = Number To Boolean Array(number="IRQ.DIO_B_7:0.ENA") -> (Boolean array=w358:bool[])
    n202 = Number To Boolean Array(number="IRQ.DIO_B_7:0.RISE") -> (Boolean array=w349:bool[])
    n203 = Number To Boolean Array(number="IRQ.DIO_B_7:0.FALL") -> (Boolean array=w344:bool[])
    n204 = Index Array(array=w358) -> (element #1=w359:bool, element #2=w357:bool, element #3=w356:bool, element #4=w355:bool)  [unwired: 4 in]
    n205 = Index Array(array=w349) -> (element #1=w348:bool, element #2=w350:bool, element #3=w351:bool, element #4=w352:bool)  [unwired: 4 in]
    n206 = Index Array(array=w344) -> (element #1=w345:bool, element #2=w343:bool, element #3=w342:bool, element #4=w341:bool)  [unwired: 4 in]
    n207 = Build Array(w359, w357, w356, w355) -> (w360:bool[])
    n208 = Build Array(w348, w350, w351, w352) -> (w347:bool[])
    n209 = Build Array(w345, w343, w342, w341) -> (w346:bool[])
    n210 = Build Array("IRQ.DIO_B_0.CNT", "IRQ.DIO_B_1.CNT", "IRQ.DIO_B_2.CNT", "IRQ.DIO_B_3.CNT") -> (w367:u32[])
    n211 = Build Array("IRQ.DIO_B_0.NO", "IRQ.DIO_B_1.NO", "IRQ.DIO_B_2.NO", "IRQ.DIO_B_3.NO") -> (w362:u8[])
    n212 = Boolean Array To Number(Boolean array=w360) -> (number=w353:fxp<+,4,4>)
    n213 = Boolean Array To Number(Boolean array=w347) -> (number=w338:fxp<+,4,4>)
    n214 = Boolean Array To Number(Boolean array=w346) -> (number=w337:fxp<+,4,4>)
    n215 = call "DIO IRQ 4-bit.vi"("IRQ NO"=w362, "IRQ CNT"=w367, "FIFO In"=w361, "IRQ.FALL"=w337, "IRQ.RISE"=w338, "IRQ.ENA"=w353, "IN 3:0"=w372) -> ()  [unwired: 5 in]
    n216 = call "Split HDC Bank2 DIO.vi"("IN 7:0"="DIO.B_15:8.OUT") -> ("OUT 5"=w378:bool, "OUT 7:6"=w402:fxp<+,2,2>, "OUT 4:3"=w380:fxp<+,2,2>, "OUT 2"=w382:bool, "OUT 0"=w386:bool, "OUT 1"=w385:bool)  [unwired: 2 in]
    n217 = call "Split HDC Bank2 DIO.vi"("IN 7:0"="DIO.B_15:8.DIR") -> ("OUT 5"=w377:bool, "OUT 7:6"=w401:fxp<+,2,2>, "OUT 4:3"=w379:fxp<+,2,2>, "OUT 2"=w381:bool, "OUT 0"=w384:bool, "OUT 1"=w383:bool)  [unwired: 2 in]
    n218 = call "DIO_PWM.vi"("DIO.OUT"=w386, "DIO.DIR"=w384, "PWM.CS"="PWM.B_0.CS", "PWM.CNFG"="PWM.B_0.CNFG", "PWM.CMP"="PWM.B_0.CMP", "PWM.MAX"="PWM.B_0.MAX", "DIO/PWM"=refnum<k21> "MXP/DIO8", "SELECT"=w396) -> ("DIO.IN"=w391:bool, "PWM.CNTR"=→"PWM.B_0.CNTR":u16)  [unwired: 10 in]
    n219 = call "DIO_PWM.vi"("DIO.OUT"=w385, "DIO.DIR"=w383, "PWM.CS"="PWM.B_1.CS", "PWM.CNFG"="PWM.B_1.CNFG", "PWM.CMP"="PWM.B_1.CMP", "PWM.MAX"="PWM.B_1.MAX", "DIO/PWM"=refnum<k21> "MXP/DIO9", "SELECT"=w395) -> ("DIO.IN"=w390:bool, "PWM.CNTR"=→"PWM.B_1.CNTR":u16)  [unwired: 10 in]
    n220 = call "DIO_PWM.vi"("DIO.OUT"=w382, "DIO.DIR"=w381, "PWM.CS"="PWM.B_2.CS", "PWM.CNFG"="PWM.B_2.CNFG", "PWM.CMP"="PWM.B_2.CMP", "PWM.MAX"="PWM.B_2.MAX", "DIO/PWM"=refnum<k21> "MXP/DIO10", "SELECT"=w394) -> ("DIO.IN"=w389:bool, "PWM.CNTR"=→"PWM.B_2.CNTR":u16)  [unwired: 10 in]
    n221 = call "DIO_Encoder.vi"("DIO.1:0.OUT"=w380, "DIO.1:0.DIR"=w379, "QE.CNFG"="ENC.B.CNFG", "DIO.1/QE.B"=refnum<k21> "MXP/DIO12", "SELECT"=w393, "DIO.0/QE.A"=refnum<k21> "MXP/DIO11") -> ("DIO.1:0.IN"=w388:fxp<+,2,2>, "QE.CNTR"=→"ENC.B.CNTR":u32, "QE.STAT"=→"ENC.B.STAT":u8)  [unwired: 11 in]
    n222 = call "DIO 1-bit.vi"("DIR"=w377, "OUT"=w378, "DIO Refnum"=refnum<k21> "MXP/DIO13") -> ("IN"=w387:bool)  [unwired: 8 in]
    n223 = call "DIO_I2C.vi"("DIO.1:0.OUT"=w402, "DIO.1:0.DIR"=w401, "I2C.CNFG"="I2C.B.CNFG", "I2C.CNTL"="I2C.B.CNTL", "I2C.ADDR"="I2C.B.ADDR", "I2C.DATO"="I2C.B.DATO", "DIO.1/I2C.SDA"=refnum<k21> "MXP/DIO15" ("DIO.1/I2C.SCL"), "I2C.CNTR"="I2C.B.CNTR", "DIO.0/I2C.SCL"=refnum<k21> "MXP/DIO14" ("DIO.0/I2C.SDA"), "Execute?"="I2C.B.GO", "SELECT"=w392) -> ("DIO.1:0.IN"=w399:fxp<+,2,2>, "I2C.DATI"=→"I2C.B.DATI":u8, "I2C.STAT"=→"I2C.B.STAT":u8)  [unwired: 6 in]
    n224 = call "Join HDC Bank2 DIO.vi"("IN 7:6"=w399, "IN 5"=w387, "IN 4:3"=w388, "IN 0"=w391, "IN 2"=w389, "IN 1"=w390) -> ("OUT 7:0"=→"DIO.B_15:8.IN":u8)  [unwired: 4 in]
  }
  n225 = while {
    stop <- FALSE stop-if-true
    # "Connector A SPI SCTL Interrupt Buffer"
    n226 = feedback #4(u8 0 ("Element")) -> (w466:u8)
    n227 = feedback #5(FALSE ("Timed Out?")) -> (w470:bool)
    n228 = case shown="False" w470 {
      tunnel: [w472 w474] -> w467
      tunnel: w466 -> [_ w474]
      frame False {
        n229 = xnode ("FIFO Method Node")("Timeout"=-1) -> ("Element"=w472:u8)  [unwired: 1 in, 2 out]
      }
      frame True {
      }
    }
    n230 = feedback-in #4(w467) -> ()
    n231 = xnode ("FIFO Method Node")("Element"=w467, "Timeout"=0) -> ("Timed Out?"=w468:bool)  [unwired: 1 in, 1 out]
    n232 = feedback-in #5(w468) -> ()
  }
  n233 = while {
    stop <- FALSE stop-if-true
    # "Connector A DIO SCTL Interrupt Buffer"
    n234 = feedback #6(u8 0 ("Element")) -> (w477:u8)
    n235 = feedback #7(FALSE ("Timed Out?")) -> (w481:bool)
    n236 = case shown="False" w481 {
      tunnel: [w483 w485] -> w478
      tunnel: w477 -> [_ w485]
      frame False {
        n237 = xnode ("FIFO Method Node")("Timeout"=-1) -> ("Element"=w483:u8)  [unwired: 1 in, 2 out]
      }
      frame True {
      }
    }
    n238 = feedback-in #6(w478) -> ()
    n239 = xnode ("FIFO Method Node")("Element"=w478, "Timeout"=0) -> ("Timed Out?"=w479:bool)  [unwired: 1 in, 1 out]
    n240 = feedback-in #7(w479) -> ()
  }
  n241 = node-c288(w18) -> ()
  n242 = node-c288() -> (w17:T5)  [unwired: 1 in]
  n243 = timed-loop {
    timing: w17 -> [_]
    timing-out: [_] -> w16
    stop <- FALSE stop-if-true
    # "Detta ska vara dio4"
    # "DIO"
    n244 = call "Split HDC Bank3 DIO.vi"("IN 7:0"="DIO.DIO_7:0.OUT") -> ("OUT 1:0"=w501:fxp<+,2,2>, "OUT 3:2"=w500:fxp<+,2,2>, "OUT 5:4"=w499:fxp<+,2,2>, "OUT 7:6"=w491:fxp<+,2,2>)
    n245 = call "Split HDC Bank3 DIO.vi"("IN 7:0"="DIO.DIO_7:0.DIR") -> ("OUT 1:0"=w497:fxp<+,2,2>, "OUT 3:2"=w496:fxp<+,2,2>, "OUT 5:4"=w495:fxp<+,2,2>, "OUT 7:6"=w490:fxp<+,2,2>)
    n246 = Number To Boolean Array(number="SYS.SELECTDIO") -> (Boolean array=w532:bool[])
    n247 = Index Array(array=w532) -> (element #1=w531:bool, element #2=w528:bool, element #3=w519:bool, element #4=w508:bool, element #5=w507:bool)  [unwired: 5 in]
    n248 = call "DIO_Encoder.vi"("DIO.1:0.OUT"=w491, "DIO.1:0.DIR"=w490, "QE.CNFG"="ENC.DIO_3.CNFG", "DIO.1/QE.B"=refnum<k21> "DIO/DIO7" ("DIO Refnum"), "SELECT"=w508, "DIO.0/QE.A"=refnum<k21> "DIO/DIO6" ("DIO Refnum")) -> ("DIO.1:0.IN"=w489:fxp<+,2,2>, "QE.CNTR"=→"ENC.DIO_3.CNTR":u32, "QE.STAT"=→"ENC.DIO_3.STAT":u8)  [unwired: 11 in]
    n249 = call "DIO_Encoder.vi"("DIO.1:0.OUT"=w501, "DIO.1:0.DIR"=w497, "QE.CNFG"="ENC.DIO_0.CNFG", "DIO.1/QE.B"=refnum<k21> "DIO/DIO1" ("DIO Refnum"), "SELECT"=w531, "DIO.0/QE.A"=refnum<k21> "DIO/DIO0" ("DIO Refnum")) -> ("DIO.1:0.IN"=w506:fxp<+,2,2>, "QE.CNTR"=→"ENC.DIO_0.CNTR":u32, "QE.STAT"=→"ENC.DIO_0.STAT":u8)  [unwired: 11 in]
    n250 = call "DIO_Encoder.vi"("DIO.1:0.OUT"=w500, "DIO.1:0.DIR"=w496, "QE.CNFG"="ENC.DIO_1.CNFG", "DIO.1/QE.B"=refnum<k21> "DIO/DIO3" ("DIO Refnum"), "SELECT"=w528, "DIO.0/QE.A"=refnum<k21> "DIO/DIO2" ("DIO Refnum")) -> ("DIO.1:0.IN"=w505:fxp<+,2,2>, "QE.CNTR"=→"ENC.DIO_1.CNTR":u32, "QE.STAT"=→"ENC.DIO_1.STAT":u8)  [unwired: 11 in]
    n251 = call "DIO_Encoder.vi"("DIO.1:0.OUT"=w499, "DIO.1:0.DIR"=w495, "QE.CNFG"="ENC.DIO_2.CNFG", "DIO.1/QE.B"=refnum<k21> "DIO/DIO5" ("DIO Refnum"), "SELECT"=w519, "DIO.0/QE.A"=refnum<k21> "DIO/DIO2" ("DIO Refnum")) -> ("DIO.1:0.IN"=w504:fxp<+,2,2>, "QE.CNTR"=→"ENC.DIO_2.CNTR":u32, "QE.STAT"=→"ENC.DIO_2.STAT":u8)  [unwired: 11 in]
    n252 = call "Join HDC Bank3 DIO.vi"("IN 7:6"=w489, "IN 5:4"=w504, "IN 3:2"=w505, "IN 1:0"=w506) -> ("OUT 7:0"=→"DIO.DIO_7:0.IN":u8)
    n253 = call "Split HDC Bank3 DIO.vi"("IN 7:0"="DIO.DIO_9:8.OUT") -> ("OUT 1:0"=w488:fxp<+,2,2>)  [unwired: 3 out]
    n254 = call "Split HDC Bank3 DIO.vi"("IN 7:0"="DIO.DIO_9:8.DIR") -> ("OUT 1:0"=w487:fxp<+,2,2>)  [unwired: 3 out]
    n255 = call "DIO_Encoder.vi"("DIO.1:0.OUT"=w488, "DIO.1:0.DIR"=w487, "QE.CNFG"="ENC.DIO_4.CNFG", "DIO.1/QE.B"=refnum<k21> "DIO/DIO9" ("DIO Refnum"), "SELECT"=w507, "DIO.0/QE.A"=refnum<k21> "DIO/DIO8" ("DIO Refnum")) -> ("DIO.1:0.IN"=w486:fxp<+,2,2>, "QE.CNTR"=→"ENC.DIO_4.CNTR":u32, "QE.STAT"=→"ENC.DIO_4.STAT":u8)  [unwired: 11 in]
    n256 = call "Join HDC Bank3 DIO.vi"("IN 1:0"=w486) -> ("OUT 7:0"=→"DIO.DIO_9:8.IN":u8)  [unwired: 3 in]
  }
  n257 = node-c288(w16) -> ()
  n258 = disable-structure shown="Disabled" {
    frame Disabled {
      # "DONT USE PWN 1, IT IS CONNECTED ON THREE OUTS"
      n259 = node-c288() -> (w543:T5)  [unwired: 1 in]
      n260 = timed-loop {
        timing: w543 -> [_]
        timing-out: [_] -> w542
        stop <- FALSE stop-if-true
        # "PWM1 were PWM8"
        # "First PWM1 were PWM0"
        # "PWM"
        n261 = call "PWM (Single Output).vi"("Clock Select"="PWM.PWM_0.CS", "Counter Control"="PWM.PWM_0.CNFG", "Output Compare Value"="PWM.PWM_0.CMP", "Max Counter Value"="PWM.PWM_0.MAX") -> ("Output"=w599:bool, "Counter Value"=→"PWM.PWM_0.CNTR":u16)  [unwired: 6 in]
        n262 = call "PWM (Single Output).vi"("Clock Select"="PWM.PWM_1.CS", "Counter Control"="PWM.PWM_1.CNFG", "Output Compare Value"="PWM.PWM_1.CMP", "Max Counter Value"="PWM.PWM_1.MAX") -> ("Output"=w593:bool, "Counter Value"=→"PWM.PWM_1.CNTR":u16)  [unwired: 6 in]
        n263 = call "PWM (Single Output).vi"("Clock Select"="PWM.PWM_2.CS", "Counter Control"="PWM.PWM_2.CNFG", "Output Compare Value"="PWM.PWM_2.CMP", "Max Counter Value"="PWM.PWM_2.MAX") -> ("Output"=w577:bool, "Counter Value"=→"PWM.PWM_2.CNTR":u16)  [unwired: 6 in]
        n264 = call "PWM (Single Output).vi"("Clock Select"="PWM.PWM_3.CS", "Counter Control"="PWM.PWM_3.CNFG", "Output Compare Value"="PWM.PWM_3.CMP", "Max Counter Value"="PWM.PWM_3.MAX") -> ("Output"=w576:bool, "Counter Value"=→"PWM.PWM_3.CNTR":u16)  [unwired: 6 in]
        n265 = call "PWM (Single Output).vi"("Clock Select"="PWM.PWM_4.CS", "Counter Control"="PWM.PWM_4.CNFG", "Output Compare Value"="PWM.PWM_4.CMP", "Max Counter Value"="PWM.PWM_4.MAX") -> ("Output"=w575:bool, "Counter Value"=→"PWM.PWM_4.CNTR":u16)  [unwired: 6 in]
        n266 = xnode "FPGA I/O Node"("PWM/PWM1"=w599, "PWM/PWM1"=w593, "PWM/PWM2"=w577, "PWM/PWM3"=w576, "PWM/PWM4"=w575) -> ()  [unwired: 5 in, 5 out]
        n267 = call "PWM (Single Output).vi"("Clock Select"="PWM.PWM_5.CS", "Counter Control"="PWM.PWM_5.CNFG", "Output Compare Value"="PWM.PWM_5.CMP", "Max Counter Value"="PWM.PWM_5.MAX") -> ("Output"=w550:bool, "Counter Value"=→"PWM.PWM_5.CNTR":u16)  [unwired: 6 in]
        n268 = call "PWM (Single Output).vi"("Clock Select"="PWM.PWM_6.CS", "Counter Control"="PWM.PWM_6.CNFG", "Output Compare Value"="PWM.PWM_6.CMP", "Max Counter Value"="PWM.PWM_6.MAX") -> ("Output"=w556:bool, "Counter Value"=→"PWM.PWM_6.CNTR":u16)  [unwired: 6 in]
        n269 = call "PWM (Single Output).vi"("Clock Select"="PWM.PWM_7.CS", "Counter Control"="PWM.PWM_7.CNFG", "Output Compare Value"="PWM.PWM_7.CMP", "Max Counter Value"="PWM.PWM_7.MAX") -> ("Output"=w572:bool, "Counter Value"=→"PWM.PWM_7.CNTR":u16)  [unwired: 6 in]
        n270 = call "PWM (Single Output).vi"("Clock Select"="PWM.PWM_8.CS", "Counter Control"="PWM.PWM_8.CNFG", "Output Compare Value"="PWM.PWM_8.CMP", "Max Counter Value"="PWM.PWM_8.MAX") -> ("Output"=w573:bool, "Counter Value"=→"PWM.PWM_8.CNTR":u16)  [unwired: 6 in]
        n271 = call "PWM (Single Output).vi"("Clock Select"="PWM.PWM_9.CS", "Counter Control"="PWM.PWM_9.CNFG", "Output Compare Value"="PWM.PWM_9.CMP", "Max Counter Value"="PWM.PWM_9.MAX") -> ("Output"=w574:bool, "Counter Value"=→"PWM.PWM_9.CNTR":u16)  [unwired: 6 in]
        n272 = xnode "FPGA I/O Node"("PWM/PWM5"=w550, "PWM/PWM6"=w556, "PWM/PWM7"=w572, "PWM/PWM1"=w573, "PWM/PWM9"=w574) -> ()  [unwired: 5 in, 5 out]
      }
      n273 = node-c288(w542) -> ()
    }
    frame Enabled {
    }
  }
  n274 = xnode "VI-Defined FIFO Configuration"() -> ("FIFO Out"=w2:refnum<k21>)
  n275 = node-c288() -> (w4:T5)  [unwired: 1 in]
  n276 = timed-loop {
    timing: w4 -> [_]
    timing-out: [_] -> w3
    tunnel: w2 -> [w611]
    stop <- FALSE stop-if-true
    # "SPI / CS DIO"
    # "SPI / SPI"
    # "SPI"
    n277 = xnode "FPGA I/O Node"() -> ("SPI MISO"=w628:bool)  [unwired: 1 in, 1 out]
    n278 = call "SPI Master.vi"("Count"="SPI.SPI.CNT", "Configuration"="SPI.SPI.CNFG", "Start?"="SPI.SPI.GO", "MISO"=w628, "Data Out"="SPI.SPI.DATO") -> ("Status"=w609:u8, "SCLK"=w622:bool, "MOSI"=w623:bool, "Data In"=→"SPI.SPI.DATI":u16)  [unwired: 3 in]
    "SPI.SPI.STAT" <- w609
    n279 = xnode "FPGA I/O Node"("SPI MOSI"=w623, "SPI CLK"=w622) -> ()  [unwired: 2 in, 2 out]
    n280 = call "SPI IRQ.vi"("SPI.A.IRQ.NO"="SPI.SPI.IRQ.NO", "SPI.STAT"=w609, "FIFO In"=w611) -> ()  [unwired: 9 in]
    n281 = call "Split HDC Bank1 DIO.vi"("IN 7:0"="DIO.SPI_CS3:0.OUT") -> ("OUT 3:0"=w618:fxp<+,4,4>)  [unwired: 2 out]
    n282 = call "Split HDC Bank1 DIO.vi"("IN 7:0"="DIO.SPI_CS3:0.DIR") -> ("OUT 3:0"=w617:fxp<+,4,4>)  [unwired: 2 out]
    n283 = call "DIO 4-bit.vi"("DIO0 Refnum"=refnum<k21> "SPI CS0", "DIO1 Refnum"=refnum<k21> "SPI CS1" ("DIO0 Refnum"), "DIO2 Refnum"=refnum<k21> "SPI CS2" ("DIO0 Refnum"), "DIR 3:0"=w617, "OUT 3:0"=w618, "DIO3 Refnum"=refnum<k21> "SPI CS3" ("DIO0 Refnum")) -> ("IN 3:0"=w616:fxp<+,4,4>)  [unwired: 5 in]
    n284 = call "Join HDC Bank1 DIO.vi"("IN 3:0"=w616) -> ("OUT 7:0"=→"DIO.SPI_CS3:0.IN":u8)  [unwired: 2 in]
  }
  n285 = while {
    stop <- FALSE stop-if-true
    # "Connector SPI SPI SCTL Interrupt Buffer"
    n286 = feedback #8(u8 0 ("Element")) -> (w635:u8)
    n287 = feedback #9(FALSE ("Timed Out?")) -> (w639:bool)
    n288 = case shown="False" w639 {
      tunnel: [w641 w643] -> w636
      tunnel: w635 -> [_ w643]
      frame False {
        n289 = xnode ("FIFO Method Node")("Timeout"=-1) -> ("Element"=w641:u8)  [unwired: 1 in, 2 out]
      }
      frame True {
      }
    }
    n290 = feedback-in #8(w636) -> ()
    n291 = xnode ("FIFO Method Node")("Element"=w636, "Timeout"=0) -> ("Timed Out?"=w637:bool)  [unwired: 1 in, 1 out]
    n292 = feedback-in #9(w637) -> ()
  }
  n293 = node-c288(w3) -> ()
  n294 = disable-structure shown="Disabled" {
    frame Disabled {
      n295 = node-c288() -> (w645:T5)  [unwired: 1 in]
      n296 = timed-loop {
        timing: w645 -> [_]
        timing-out: [_] -> w644
        stop <- FALSE stop-if-true
        # "I2C"
        n297 = call "DIO_I2C.vi"("I2C.CNFG"="I2C.I2C.CNFG", "I2C.CNTL"="I2C.I2C.CNTL", "I2C.ADDR"="I2C.I2CADDR", "I2C.DATO"="I2C.I2C.DATO", "DIO.1/I2C.SDA"=refnum<k21> "I2C SDA" ("FPGA I/O In"), "I2C.CNTR"="I2C.I2C.CNTR", "DIO.0/I2C.SCL"=refnum<k21> "I2C SCL" ("FPGA I/O In"), "Execute?"="I2C.I2C.GO", "SELECT"=TRUE) -> ("I2C.DATI"=→"I2C.I2C.DATI":u8, "I2C.STAT"=→"I2C.I2C.STAT":u8)  [unwired: 8 in, 1 out]
      }
      n298 = node-c288(w644) -> ()
    }
    frame Enabled {
    }
  }
  n299 = disable-structure shown="Disabled" {
    frame Disabled {
      n300 = node-c288() -> (w665:T5)  [unwired: 1 in]
      n301 = timed-loop {
        timing: w665 -> [_]
        timing-out: [_] -> w664
        stop <- FALSE stop-if-true
        # "Relay"
        n302 = Number To Boolean Array(number="DO.RELAY.OUT") -> (Boolean array=w680:bool[])
        n303 = Index Array(array=w680) -> (element #1=w679:bool, element #2=w678:bool, element #3=w677:bool, element #4=w676:bool, element #5=w675:bool, element #6=w674:bool, element #7=w673:bool, element #8=w672:bool)  [unwired: 8 in]
        n304 = xnode "FPGA I/O Node"("RelayFwd0"=w679, "RelayRev0"=w678, "RelayFwd1"=w677, "RelayRev1"=w676, "RelayFwd2"=w675, "RelayRev2"=w674, "RelayFwd3"=w673, "RelayRev3"=w672) -> ()  [unwired: 8 in, 8 out]
      }
      n305 = node-c288(w664) -> ()
      n306 = node-c288() -> (w663:T5)  [unwired: 1 in]
      n307 = timed-loop {
        timing: w663 -> [_]
        timing-out: [_] -> w662
        stop <- FALSE stop-if-true
        # "RSL"
        n308 = xnode "FPGA I/O Node"("RSL"="DO.RSL.OUT") -> ()  [unwired: 1 in, 1 out]
      }
      n309 = node-c288(w662) -> ()
    }
    frame Enabled {
    }
  }
